vi "ReadVolt.vi"(10 "starting address":u16, 11 "VISA resource name":refnum<visa-resource-name>) -> (0 "error out":errorcluster, 2 "value":dbl)   [LabVIEW 2024]
uses:
  <vilib>/NI/Modbus Library/API/Wrapper/Create Serial Master.vi
  <vilib>/NI/Modbus Library/API/Master/Modbus Master.lvclass
  <vilib>/NI/Modbus Library/API/Wrapper/API Main.lvlib
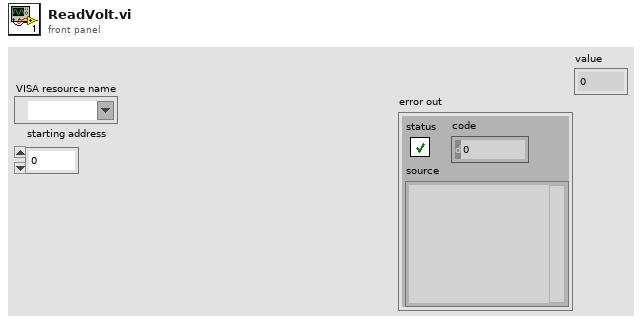
[diagram p1: front panel]
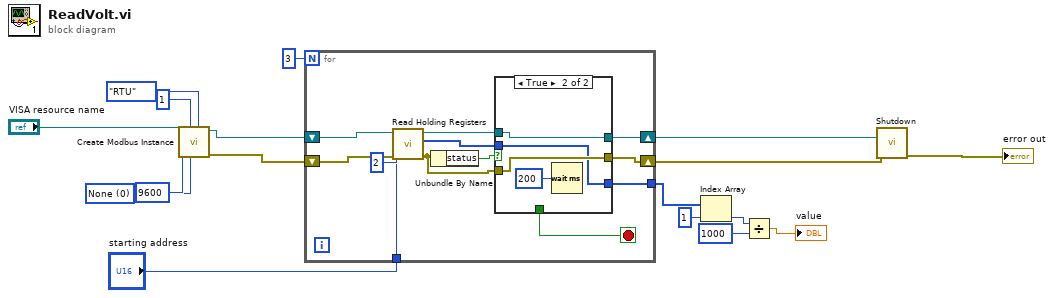
[diagram p0: block diagram]
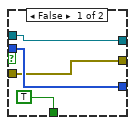
[diagram p2: hidden frame]
diagram:
  w8 = u16 0 items=["None", "Odd", "Even", "Mark", "Space"] ("parity (even)")
  n1 = call-poly <vilib>:"Create Modbus Instance.vi"("serial type"=enum16{"RTU", "ASCII"}."RTU", "parity (even)"=w8, "unit ID"=u8 1, "baud rate"=u32 9600, "VISA resource name"="VISA resource name") -> ("error out"=w12:errorcluster, "serial master instance"=w13:refnum<class "Modbus Master.lvclass">)  [unwired: 5 in]
  n2 = for {
    N: 3 -> [_]
    tunnel: "starting address" -> [w26]
    shift-right: [w23] -> w11
    shift-left: w13 -> [w29]
    shift-right: [w18] -> w10
    shift-left: w12 -> [w28]
    tunnel: [w21] -> w1
    stop <- w20 stop-if-true
    n3 = call-dynamic "Read Holding Registers.vi"("error in"=w28, "number of inputs"=u16 2, "starting address"=w26, "Modbus master in"=w29) -> ("error out"=w19:errorcluster, "register values"=w22:u16[], "Modbus master out"=w24:refnum<class "Modbus Master.lvclass">)  [unwired: 5 in]
    n4 = Unbundle By Name(w19) -> ("status"=w25:bool)
    n5 = case shown="True" w25 {
      tunnel: w24 -> [w33 w36]
      tunnel: [w33 w36] -> w23
      tunnel: w22 -> [w32 w34]
      tunnel: [w32 w34] -> w21
      tunnel: [TRUE _] -> w20
      tunnel: w19 -> [w30 w35]
      tunnel: [w30 w35] -> w18
      frame False {
      }
      frame True {
        n6 = Wait (ms)(milliseconds to wait=u32 200) -> ()  [unwired: 1 out]
      }
    }
  }
  n7 = Index Array(array=w1, index=1) -> (element=w5:u16)
  n8 = Divide(x=w5, y=u16 1000) -> (x/y=→"value":dbl)
  n9 = call-dynamic "Shutdown.vi"("error in"=w10, "Modbus master in"=w11) -> ("error out"=→"error out":errorcluster)  [unwired: 9 in]
